vi "Report_generator.vi"() -> ()   [LabVIEW 2022 SP3]
uses:
  <vilib>/Utility/NIReport.llb/Report Type.ctl
  <vilib>/Utility/NIReport.llb/Append Report Text (str wrap).vi
  <vilib>/printing/ReportDocExtensions.llb/Append VI Icon to Report (refnum).vi
  <vilib>/printing/ReportDocExtensions.llb/Append VI Description to Report (refnum).vi
  <vilib>/printing/ReportDocExtensions.llb/Append Front Panel Image to Report (refnum).vi
  <vilib>/printing/ReportDocExtensions.llb/Append VI List of Controls to Report (refnum).vi
  <vilib>/printing/ReportDocExtensions.llb/Append VI List of SubVIs to Report (refnum).vi
  <vilib>/printing/ReportDocExtensions.llb/Append VI Hierarchy to Report (refnum).vi
  <vilib>/Utility/NIReport.llb/NI_report.lvclass
  <vilib>/Utility/NIReport.llb/NI_ReportGenerationCore.lvlib
panel:
  out "error out":errorcluster
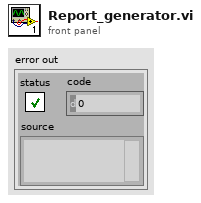
[diagram p1: front panel]
types:
  T1 = typedef "NI_ReportGenerationCore.lvlib/Report Type.ctl" = enum16{"HTML", "Word", "Excel"}
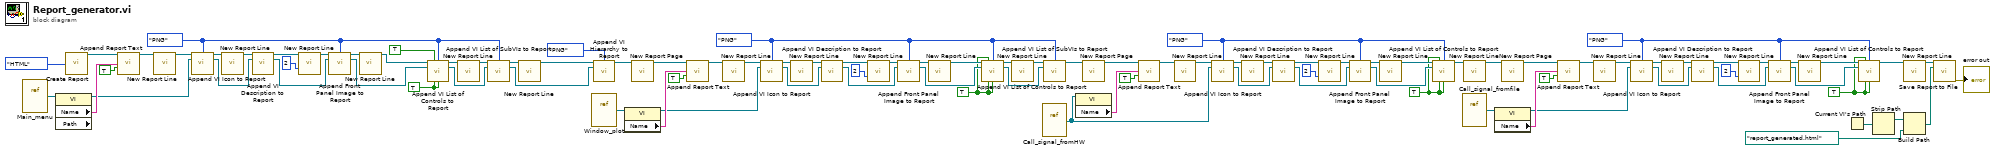
[diagram p0: block diagram]
diagram:
  w2 = enum32{"PNG", "JPEG", "GIF"}."PNG" ("image format (jpeg)")
  w10 = TRUE ("include only controls in con pane?")
  w3 = enum32{"PNG", "JPEG", "GIF"}."PNG" ("image format (jpeg)")
  w11 = TRUE ("include only controls in con pane?")
  w4 = enum32{"PNG", "JPEG", "GIF"}."PNG" ("image format (jpeg)")
  w12 = TRUE ("include only controls in con pane?")
  w5 = enum32{"PNG", "JPEG", "GIF"}."PNG" ("image format (jpeg)")
  w13 = TRUE ("include only controls in con pane?")
  n1 = vi-ref "Main_menu.vi"() -> (w72:refnum<vi>)
  n2 = property class="VI" props=["Name", "Path"](reference=w72) -> (reference out=w16:refnum<vi>, "Name"=w71:string)  [unwired: 1 in, 2 out]
  n3 = call <vilib>:"Create Report.vi"("report type"=Report_Type."HTML") -> ("report out"=w97:refnum<class "NI_report.lvclass">)  [unwired: 13 in, 1 out]
  n4 = call-poly <vilib>:"Append Report Text.vi"("report in"=w97, "text"=w71, "append on new line? (F)"=TRUE) -> ("report out"=w91:refnum<class "NI_report.lvclass">)  [unwired: 9 in, 3 out]
  n5 = call-dynamic "New Report Line.vi"("report in"=w91) -> ("report out"=w90:refnum<class "NI_report.lvclass">)  [unwired: 13 in, 1 out]
  n6 = call-poly <vilib>:"Append VI Icon to Report.vi"("report in"=w90, "image format (jpeg)"=w5, "VI"=w16) -> ("report out"=w83:refnum<class "NI_report.lvclass">, "VI out"=w89:refnum<vi>)  [unwired: 8 in, 3 out]
  n7 = call-dynamic "New Report Line.vi"("report in"=w83) -> ("report out"=w84:refnum<class "NI_report.lvclass">)  [unwired: 13 in, 1 out]
  n8 = call-poly <vilib>:"Append VI Description to Report.vi"("report in"=w84, "VI"=w89) -> ("report out"=w80:refnum<class "NI_report.lvclass">, "VI out"=w88:refnum<vi>)  [unwired: 9 in, 3 out]
  n9 = call-dynamic "New Report Line.vi"("report in"=w80, "number of lines (1)"=2) -> ("report out"=w79:refnum<class "NI_report.lvclass">)  [unwired: 12 in, 1 out]
  n10 = call-poly <vilib>:"Append Front Panel Image to Report.vi"("report in"=w79, "image format (jpeg)"=w5, "VI"=w88) -> ("report out"=w82:refnum<class "NI_report.lvclass">, "VI out"=w87:refnum<vi>)  [unwired: 8 in, 3 out]
  n11 = call-dynamic "New Report Line.vi"("report in"=w82) -> ("report out"=w81:refnum<class "NI_report.lvclass">)  [unwired: 13 in, 1 out]
  n12 = call-poly <vilib>:"Append VI List of Controls to Report.vi"("report in"=w81, "include only controls in con pane?"=TRUE, "image format (jpeg)"=w5, "VI"=w87, "include control descriptions?"=w13, "include control data types?"=w13) -> ("report out"=w77:refnum<class "NI_report.lvclass">, "VI out"=w86:refnum<vi>)  [unwired: 5 in, 3 out]
  n13 = call-dynamic "New Report Line.vi"("report in"=w77) -> ("report out"=w76:refnum<class "NI_report.lvclass">)  [unwired: 13 in, 1 out]
  n14 = call-poly <vilib>:"Append VI List of SubVIs to Report.vi"("report in"=w76, "image format (jpeg)"=w5, "VI"=w86) -> ("report out"=w75:refnum<class "NI_report.lvclass">, "VI out"=w85:refnum<vi>)  [unwired: 8 in, 3 out]
  n15 = call-dynamic "New Report Line.vi"("report in"=w75) -> ("report out"=w74:refnum<class "NI_report.lvclass">)  [unwired: 13 in, 1 out]
  n16 = vi-ref "Window_plot.vi"() -> (w52:refnum<vi>)
  n17 = call-poly <vilib>:"Append VI Hierarchy to Report.vi"("report in"=w74, "image format (jpeg)"=enum32{"PNG", "JPEG", "GIF"}."PNG", "VI"=w85) -> ("report out"=w73:refnum<class "NI_report.lvclass">)  [unwired: 8 in, 4 out]
  n18 = property class="VI"(reference=w52) -> (reference out=w17:refnum<vi>, "Name"=w70:string)  [unwired: 1 in, 1 out]
  n19 = call-dynamic "New Report Page.vi"("report in"=w73) -> ("report out"=w53:refnum<class "NI_report.lvclass">)  [unwired: 13 in, 1 out]
  n20 = call-poly <vilib>:"Append Report Text.vi"("report in"=w53, "text"=w70, "append on new line? (F)"=TRUE) -> ("report out"=w55:refnum<class "NI_report.lvclass">)  [unwired: 9 in, 3 out]
  n21 = call-dynamic "New Report Line.vi"("report in"=w55) -> ("report out"=w56:refnum<class "NI_report.lvclass">)  [unwired: 13 in, 1 out]
  n22 = call-poly <vilib>:"Append VI Icon to Report.vi"("report in"=w56, "image format (jpeg)"=w4, "VI"=w17) -> ("report out"=w62:refnum<class "NI_report.lvclass">, "VI out"=w57:refnum<vi>)  [unwired: 8 in, 3 out]
  n23 = call-dynamic "New Report Line.vi"("report in"=w62) -> ("report out"=w61:refnum<class "NI_report.lvclass">)  [unwired: 13 in, 1 out]
  n24 = call-poly <vilib>:"Append VI Description to Report.vi"("report in"=w61, "VI"=w57) -> ("report out"=w65:refnum<class "NI_report.lvclass">, "VI out"=w58:refnum<vi>)  [unwired: 9 in, 3 out]
  n25 = call-dynamic "New Report Line.vi"("report in"=w65, "number of lines (1)"=2) -> ("report out"=w66:refnum<class "NI_report.lvclass">)  [unwired: 12 in, 1 out]
  n26 = call-poly <vilib>:"Append Front Panel Image to Report.vi"("report in"=w66, "image format (jpeg)"=w4, "VI"=w58) -> ("report out"=w63:refnum<class "NI_report.lvclass">, "VI out"=w59:refnum<vi>)  [unwired: 8 in, 3 out]
  n27 = call-dynamic "New Report Line.vi"("report in"=w63) -> ("report out"=w64:refnum<class "NI_report.lvclass">)  [unwired: 13 in, 1 out]
  n28 = call-poly <vilib>:"Append VI List of Controls to Report.vi"("report in"=w64, "include only controls in con pane?"=w12, "image format (jpeg)"=w4, "VI"=w59, "include control descriptions?"=w12, "include control data types?"=w12) -> ("report out"=w68:refnum<class "NI_report.lvclass">, "VI out"=w60:refnum<vi>)  [unwired: 5 in, 3 out]
  n29 = call-dynamic "New Report Line.vi"("report in"=w68) -> ("report out"=w69:refnum<class "NI_report.lvclass">)  [unwired: 13 in, 1 out]
  n30 = vi-ref "Call_signal_fromHW.vi"() -> (w36:refnum<vi>)
  n31 = call-poly <vilib>:"Append VI List of SubVIs to Report.vi"("report in"=w69, "image format (jpeg)"=w4, "VI"=w60) -> ("report out"=w6:refnum<class "NI_report.lvclass">)  [unwired: 8 in, 4 out]
  n32 = property class="VI"(reference=w36) -> ("Name"=w37:string)  [unwired: 1 in, 2 out]
  n33 = call-dynamic "New Report Page.vi"("report in"=w6) -> ("report out"=w20:refnum<class "NI_report.lvclass">)  [unwired: 13 in, 1 out]
  n34 = call-poly <vilib>:"Append Report Text.vi"("report in"=w20, "text"=w37, "append on new line? (F)"=TRUE) -> ("report out"=w50:refnum<class "NI_report.lvclass">)  [unwired: 9 in, 3 out]
  n35 = call-dynamic "New Report Line.vi"("report in"=w50) -> ("report out"=w49:refnum<class "NI_report.lvclass">)  [unwired: 13 in, 1 out]
  n36 = call-poly <vilib>:"Append VI Icon to Report.vi"("report in"=w49, "image format (jpeg)"=w3, "VI"=w36) -> ("report out"=w44:refnum<class "NI_report.lvclass">, "VI out"=w48:refnum<vi>)  [unwired: 8 in, 3 out]
  n37 = call-dynamic "New Report Line.vi"("report in"=w44) -> ("report out"=w45:refnum<class "NI_report.lvclass">)  [unwired: 13 in, 1 out]
  n38 = call-poly <vilib>:"Append VI Description to Report.vi"("report in"=w45, "VI"=w48) -> ("report out"=w41:refnum<class "NI_report.lvclass">, "VI out"=w47:refnum<vi>)  [unwired: 9 in, 3 out]
  n39 = call-dynamic "New Report Line.vi"("report in"=w41, "number of lines (1)"=2) -> ("report out"=w40:refnum<class "NI_report.lvclass">)  [unwired: 12 in, 1 out]
  n40 = call-poly <vilib>:"Append Front Panel Image to Report.vi"("report in"=w40, "image format (jpeg)"=w3, "VI"=w47) -> ("report out"=w43:refnum<class "NI_report.lvclass">, "VI out"=w46:refnum<vi>)  [unwired: 8 in, 3 out]
  n41 = call-dynamic "New Report Line.vi"("report in"=w43) -> ("report out"=w42:refnum<class "NI_report.lvclass">)  [unwired: 13 in, 1 out]
  n42 = call-poly <vilib>:"Append VI List of Controls to Report.vi"("report in"=w42, "include only controls in con pane?"=w11, "image format (jpeg)"=w3, "VI"=w46, "include control descriptions?"=w11, "include control data types?"=w11) -> ("report out"=w38:refnum<class "NI_report.lvclass">)  [unwired: 5 in, 4 out]
  n43 = vi-ref "Call_signal_fromfile.vi"() -> (w19:refnum<vi>)
  n44 = call-dynamic "New Report Line.vi"("report in"=w38) -> ("report out"=w9:refnum<class "NI_report.lvclass">)  [unwired: 13 in, 1 out]
  n45 = property class="VI"(reference=w19) -> (reference out=w15:refnum<vi>, "Name"=w35:string)  [unwired: 1 in, 1 out]
  n46 = call-dynamic "New Report Page.vi"("report in"=w9) -> ("report out"=w18:refnum<class "NI_report.lvclass">)  [unwired: 13 in, 1 out]
  n47 = call-poly <vilib>:"Append Report Text.vi"("report in"=w18, "text"=w35, "append on new line? (F)"=TRUE) -> ("report out"=w22:refnum<class "NI_report.lvclass">)  [unwired: 9 in, 3 out]
  n48 = call-dynamic "New Report Line.vi"("report in"=w22) -> ("report out"=w23:refnum<class "NI_report.lvclass">)  [unwired: 13 in, 1 out]
  n49 = call-poly <vilib>:"Append VI Icon to Report.vi"("report in"=w23, "image format (jpeg)"=w2, "VI"=w15) -> ("report out"=w28:refnum<class "NI_report.lvclass">, "VI out"=w24:refnum<vi>)  [unwired: 8 in, 3 out]
  n50 = call-dynamic "New Report Line.vi"("report in"=w28) -> ("report out"=w27:refnum<class "NI_report.lvclass">)  [unwired: 13 in, 1 out]
  n51 = call-poly <vilib>:"Append VI Description to Report.vi"("report in"=w27, "VI"=w24) -> ("report out"=w31:refnum<class "NI_report.lvclass">, "VI out"=w25:refnum<vi>)  [unwired: 9 in, 3 out]
  n52 = call-dynamic "New Report Line.vi"("report in"=w31, "number of lines (1)"=2) -> ("report out"=w32:refnum<class "NI_report.lvclass">)  [unwired: 12 in, 1 out]
  n53 = call-poly <vilib>:"Append Front Panel Image to Report.vi"("report in"=w32, "image format (jpeg)"=w2, "VI"=w25) -> ("report out"=w29:refnum<class "NI_report.lvclass">, "VI out"=w26:refnum<vi>)  [unwired: 8 in, 3 out]
  n54 = call-dynamic "New Report Line.vi"("report in"=w29) -> ("report out"=w30:refnum<class "NI_report.lvclass">)  [unwired: 13 in, 1 out]
  n55 = Current VI's Path() -> (path=w96:path)
  n56 = call-poly <vilib>:"Append VI List of Controls to Report.vi"("report in"=w30, "include only controls in con pane?"=w10, "image format (jpeg)"=w2, "VI"=w26, "include control descriptions?"=w10, "include control data types?"=w10) -> ("report out"=w34:refnum<class "NI_report.lvclass">)  [unwired: 5 in, 4 out]
  n57 = Strip Path(path=w96) -> (stripped path=w95:path)  [unwired: 1 out]
  n58 = call-dynamic "New Report Line.vi"("report in"=w34) -> ("report out"=w14:refnum<class "NI_report.lvclass">)  [unwired: 13 in, 1 out]
  n59 = Build Path(base path=w95, name or relative path=path "report_generated.html") -> (appended path=w93:path)
  n60 = call-dynamic "Save Report to File.vi"("report in"=w14, "report file path"=w93) -> ("error out"=→"error out":errorcluster)  [unwired: 12 in, 1 out]
